vi "remotecall_2.vi"() -> ()   [LabVIEW 2015]
panel:
  in  "Fun":enum16{"Count", "Init"}(ring)
  in  "timeout ms (60000)":i32=60000
  in  "machine name (\"\":  open local reference)":string="127.0.0.1"
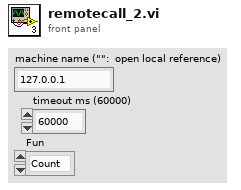
[diagram p1: front panel]
types:
  T1 = enum32{"Invalid", "Standard", "Closed", "Hidden", "Minimized", "Maximized"}
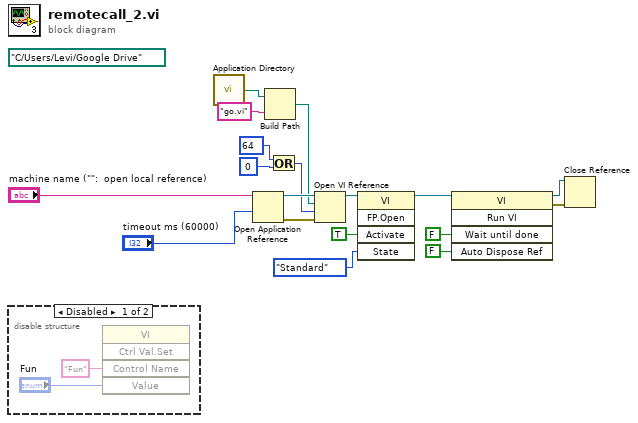
[diagram p0: block diagram]
diagram:
  (unwired) path "C:/Users/Levi/Google Drive" ("vi path")
  n1 = disable-structure shown="Disabled" {
    frame Disabled {
      n2 = invoke class="VI" method="Ctrl Val.Set"("Control Name"="Fun", "Value"="Fun") -> ()  [unwired: 3 in, 5 out]
    }
    frame Enabled {
    }
  }
  n3 = call <vilib>:"Application Directory.vi"() -> ("Application Directory"=w8:path)
  n4 = Open Application Reference(9:"timeout ms (60000)", 11:"machine name (\"\":  open local reference)") -> (0:w16:errorcluster, 3:w17:refnum<vi>)  [unwired: 2 in]
  n5 = Build Path(base path=w8, name or relative path="go.vi") -> (appended path=w9:path)
  n6 = Or(x=64 ("options"), y=0 ("options")) -> (x .or. y?=w5:i32)
  n7 = Open VI Reference(application reference (local)=w17, vi path=w9, options=w5, error in (no error)=w16) -> (vi reference=w4:refnum<vi>)  [unwired: 2 in, 1 out]
  n8 = invoke class="VI" method="FP.Open"(reference=w4, "Activate"=TRUE ("Activate?"), "State"=T1."Standard") -> (reference out=w3:refnum<vi>)  [unwired: 2 in, 4 out]
  n9 = invoke class="VI" method="Run VI"(reference=w3, "Wait until done"=FALSE ("Wait Until Done"), "Auto Dispose Ref"=FALSE ("Auto Dispose Reference")) -> (reference out=w12:refnum<vi>, error out=w11:errorcluster)  [unwired: 2 in, 3 out]
  n10 = Close Reference(reference=w12, error in (no error)=w11) -> ()  [unwired: 1 out]
